vi "validate_position_v0.01.vi"(0 "valve Time Cluster":T1, 1 "which manipulator":T5(ring), 2 "Which Position to use for Experiment":T4(ring), 3 "data in":T2={"daq_ao 1"="Dev1/ao0", "daq_ai 1"="Dev1/ai0", "experiment day folder"=path "D:/DATA/8-27-15 save func testing/test.lvm", "Multiclamp init error"=0, "Multiclamp Handle Out"=0, "sampling rate (Hz)"=10000, "trial name"=""}, 7 "controls array in":refnum<vi>[](array[refnum]), 9 "time to wait for solution change (min)":dbl=2.5 min=0.0 step=0.01, 11 "error in":errorcluster, 12 "common cluster":T7, 13 "individual controls in":T6) -> (4 "output cluster":T3={"daq_ao 2"="", "Duration (s)"=0.0, "Sample Freq (Hz)"=0.0, "Phase"=0.0, "Duty Cycle"=0.0, "Jump Filter Freq (Hz)"=0.0, "Number of Replicates"=1} {"Number of Replicates" min=1 max=10}, 6 "output waveform":waveform(dbl)(graph), 8 "protocol response":waveform(dbl)[](graph) caption="Memtest", 10 "control array out":refnum<vi>[](array[refnum]), 15 "error out":errorcluster)   [LabVIEW 2019]
uses:
  pipette cleaning/pressure box/cleaning_soft/controls/actuator_type.ctl
  pipette cleaning/pressure box/cleaning_soft/controls/actuator_cluster.ctl
  machine_vision/coordinate model vis/transform_properties_actuators.ctl
  machine_vision/controls/transform_cluster_actuator.ctl
  controls/NH_method.ctl
  pipette cleaning/pressure box/cleaning_soft/controls/pressure_box_type.ctl
  pipette cleaning/pressure box/cleaning_soft/controls/pressure_box_control.ctl
  multipatch/controls/multipatch_common_controls_v4.ctl
  controls/memtest_def.ctl
  multipatch/controls/multipatch_individual_controls_v5.ctl
  Controls/Data.ctl
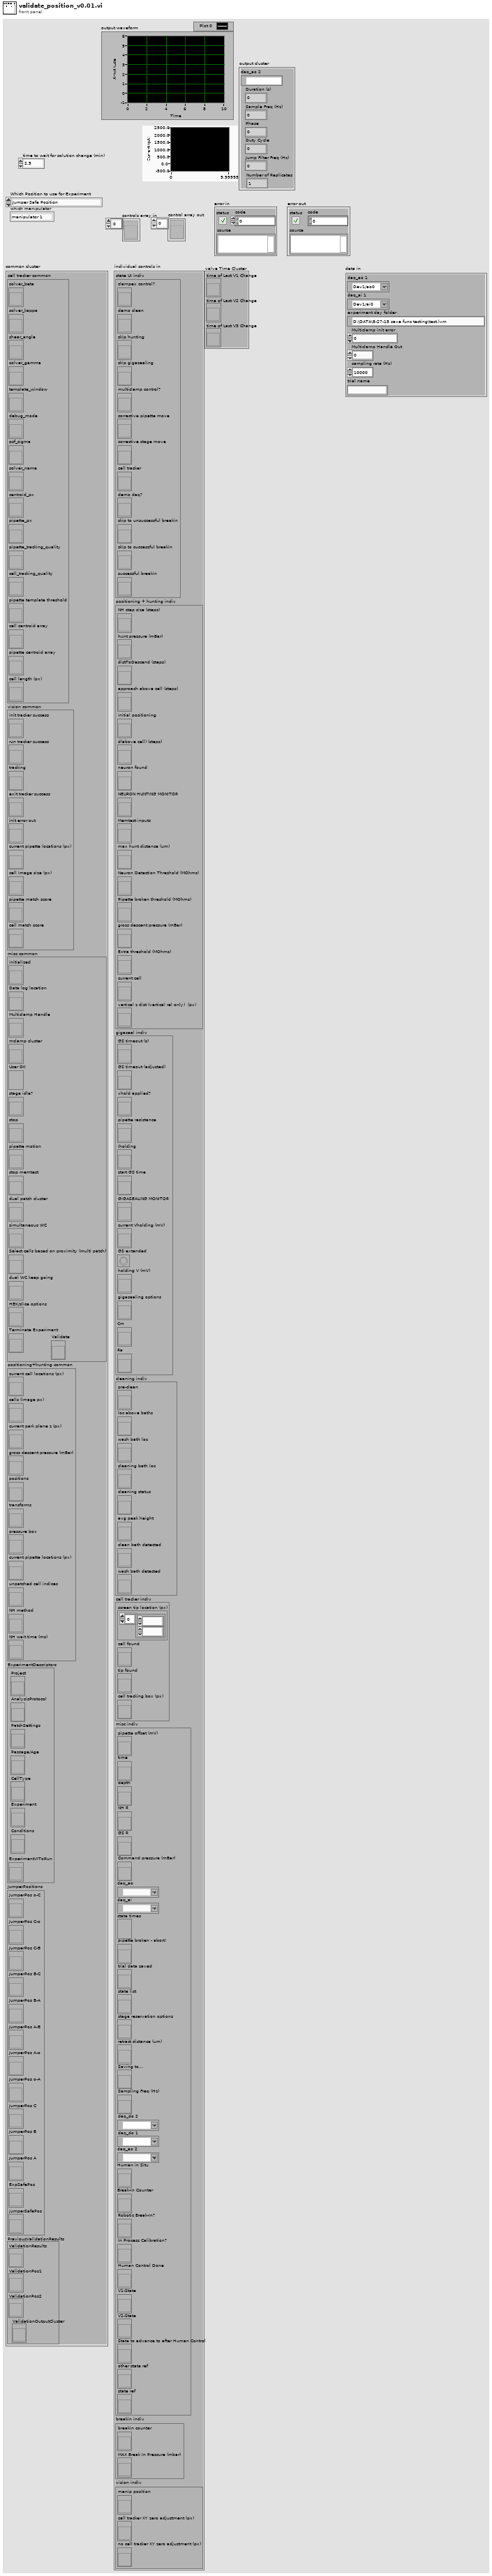
[diagram p1: front panel]
types:
  T1 = cluster{"time of Last V1 Change":refnum<vi>, "time of Last V2 Change":refnum<vi>, "time of Last V3 Change":refnum<vi>}
  T2 = typedef "Data.ctl" = cluster{"daq_ao 1":tag, "daq_ai 1":tag, "experiment day folder":path, "Multiclamp init error":i32, "Multiclamp Handle Out":u32, "sampling rate (Hz)":i32, "trial name":string}
  T3 = cluster{"daq_ao 2":tag, "Duration (s)":dbl, "Sample Freq (Hz)":dbl, "Phase":dbl, "Duty Cycle":dbl, "Jump Filter Freq (Hz)":dbl, "Number of Replicates":i16}
  T4 = enum16{"Jumper Safe Position", "Experiment Safe Position", "Jumper Position A", "Jumper Position B", "Jumper Position C", "Jumper Position o-A", "Jumper Position A-o", "Jumper Position A-B", "Jumper Position B-A", "Jumper Position B-C", "Jumper Position C-B", "Jumper Position C-o", "Jumper Position o-C"}
  T5 = enum16{"manipulator 1", "manipulator 2", "manipulator 3", "manipulator 4"}
  T6 = typedef "multipatch_individual_controls_v5.ctl" = cluster{"state UI indiv":cluster{"clampex control?":refnum<vi>, "demo clean":refnum<vi>, "skip hunting":refnum<vi>, "skip gigasealing":refnum<vi>, "multiclamp control?":refnum<vi>, "corrective pipette move":refnum<vi>, "corrective stage move":refnum<vi>, "cell tracker":refnum<vi>, "demo daq?":refnum<vi>, "skip to unsuccessful breakin":refnum<vi>, "skip to successful breakin":refnum<vi>, "successful breakin":refnum<vi>}, "positioning + hunting indiv":cluster{"NH step size (steps)":refnum<vi>, "hunt pressure (mBar)":refnum<vi>, "distToDescend (steps)":refnum<vi>, "approach above cell (steps)":refnum<vi>, "initial positioning":refnum<vi>, "d(above cell) (steps)":refnum<vi>, "neuron found":refnum<vi>, "NEURON HUNTING MONITOR":refnum<vi>, "Memtest inputs":refnum<vi>, "max hunt distance (um)":refnum<vi>, "Neuron Detection Threshold (MOhms)":refnum<vi>, "Pipette broken threshold (MOhms)":refnum<vi>, "gross descent pressure (mBar)":refnum<vi>, "Extra threshold (MOhms)":refnum<vi>, "current cell":refnum<vi>, "vertical z dist (vertical rel only)  (px)":refnum<vi>}, "gigaseal indiv":cluster{"GS timeout (s)":refnum<vi>, "GS timeout (adjusted)":refnum<vi>, "vhold applied?":refnum<vi>, "pipette resistance":refnum<vi>, "Iholding":refnum<vi>, "start GS time":refnum<vi>, "GIGASEALING MONITOR":refnum<vi>, "current Vholding (mV)":refnum<vi>, "GS extended":refnum<vi>, "holding V (mV)":refnum<vi>, "gigasealing options":refnum<vi>, "Cm":refnum<vi>, "Ra ":refnum<vi>}, "cleaning indiv":cluster{"pre-clean":refnum<vi>, "loc above baths":refnum<vi>, "wash bath loc":refnum<vi>, "cleaning bath loc":refnum<vi>, "cleaning status":refnum<vi>, "avg peak height":refnum<vi>, "clean bath detected":refnum<vi>, "wash bath detected":refnum<vi>}, "cell tracker indiv":cluster{"screen tip location (px)":refnum<vi>, "cell found":refnum<vi>, "tip found":refnum<vi>, "cell tracking box (px)":refnum<vi>}, "misc indiv":cluster{"pipette offset (mV)":refnum<vi>, "time":refnum<vi>, "depth":refnum<vi>, "NH R":refnum<vi>, "GS R":refnum<vi>, "Command pressure (mBar)":refnum<vi>, "daq_ao":tag, "daq_ai":tag, "state times":refnum<vi>, "pipette broken - abort!":refnum<vi>, "trial data saved":refnum<vi>, "state list":refnum<vi>, "stage reservation options":refnum<vi>, "retract distance (um)":refnum<vi>, "Saving to...":refnum<vi>, "Sampling Freq (Hz)":refnum<vi>, "daq_do 2":tag, "daq_do 1":tag, "daq_ao 2":tag, "Human in Situ":refnum<vi>, "Break-In Counter":refnum<vi>, "Robotic Break-In?":refnum<vi>, "In Process Calibration?":refnum<vi>, "Human Control Done":refnum<vi>, "V1-State":refnum<vi>, "V2-State":refnum<vi>, "State to advance to after Human Control":refnum<vi>, "other state ref":refnum<vi>, "state ref":refnum<vi>}, "breakin indiv":cluster{"breakin counter":refnum<vi>, "MAX Break In Pressure (mbar)":refnum<vi>}, "vision indiv":cluster{"manip position":refnum<vi>, "cell tracker XY zero adjustment (px)":refnum<vi>, "no cell tracker XY zero adjustment (px)":refnum<vi>}}
  T7 = typedef "multipatch_common_controls_v4.ctl" = cluster{"cell tracker common":cluster{"solver_beta":refnum<vi>, "solver_kappa":refnum<vi>, "shear_angle":refnum<vi>, "solver_gamma":refnum<vi>, "template_window":refnum<vi>, "debug_mode":refnum<vi>, "psf_sigma":refnum<vi>, "solver_name":refnum<vi>, "centroid_px":refnum<vi>, "pipette_px":refnum<vi>, "pipette_tracking_quality":refnum<vi>, "cell_tracking_quality":refnum<vi>, "pipette template threshold":refnum<vi>, "cell centroid array":refnum<vi>, "pipette centroid array":refnum<vi>, "cell length (px)":refnum<vi>}, "vision common":cluster{"init tracker success":refnum<vi>, "run tracker success":refnum<vi>, "tracking":refnum<vi>, "exit tracker success":refnum<vi>, "init error out":refnum<vi>, "current pipette locations (px)":refnum<vi>, "cell image size (px)":refnum<vi>, "pipette match score":refnum<vi>, "cell match score":refnum<vi>}, "misc common":cluster{"initialized":refnum<vi>, "Data log location":refnum<vi>, "Multiclamp Handle":refnum<vi>, "mclamp cluster":refnum<vi>, "User OK":refnum<vi>, "stage idle?":refnum<vi>, "stop":refnum<vi>, "pipette motion":refnum<vi>, "stop memtest":refnum<vi>, "dual patch cluster":refnum<vi>, "simultaneous WC":refnum<vi>, "Select cells based on proximity (multi patch)":refnum<vi>, "dual WC keep going":refnum<vi>, "HEK/slice options":refnum<vi>, "Terminate Experiment":refnum<vi>, "Validate":refnum<vi>}, "positioning+hunting common":cluster{"current cell locations (px)":refnum<vi>, "cells (image px)":refnum<vi>, "current park plane z (px)":refnum<vi>, "gross descent pressure (mBar)":refnum<vi>, "positions":refnum<vi>, "transforms":refnum<vi>, "pressure box":refnum<vi>, "current pipette locations (px)":refnum<vi>, "unpatched cell indices":refnum<vi>, "NH method":refnum<vi>, "NH wait time (ms)":refnum<vi>}, "ExperimentDescriptors":cluster{"Project":refnum<vi>, "AnalysisProtocol":refnum<vi>, "PatchSettings":refnum<vi>, "Passage/Age":refnum<vi>, "CellType":refnum<vi>, "Experiment":refnum<vi>, "Conditions":refnum<vi>, "ExperimentVIToRun":refnum<vi>}, "JumperPositions":cluster{"JumperPos o-C":refnum<vi>, "JumperPos C-o":refnum<vi>, "JumperPos C-B":refnum<vi>, "JumperPos B-C":refnum<vi>, "JumperPos B-A":refnum<vi>, "JumperPos A-B":refnum<vi>, "JumperPos A-o":refnum<vi>, "JumperPos o-A":refnum<vi>, "JumperPos C":refnum<vi>, "JumperPos B":refnum<vi>, "JumperPos A":refnum<vi>, "ExpSafePos":refnum<vi>, "jumperSafePos":refnum<vi>}, "PreviousValidationResults":cluster{"ValidationResults":refnum<vi>, "ValidationPos1":refnum<vi>, "ValidationPos2":refnum<vi>, "ValidationOutputCluster":refnum<vi>}}
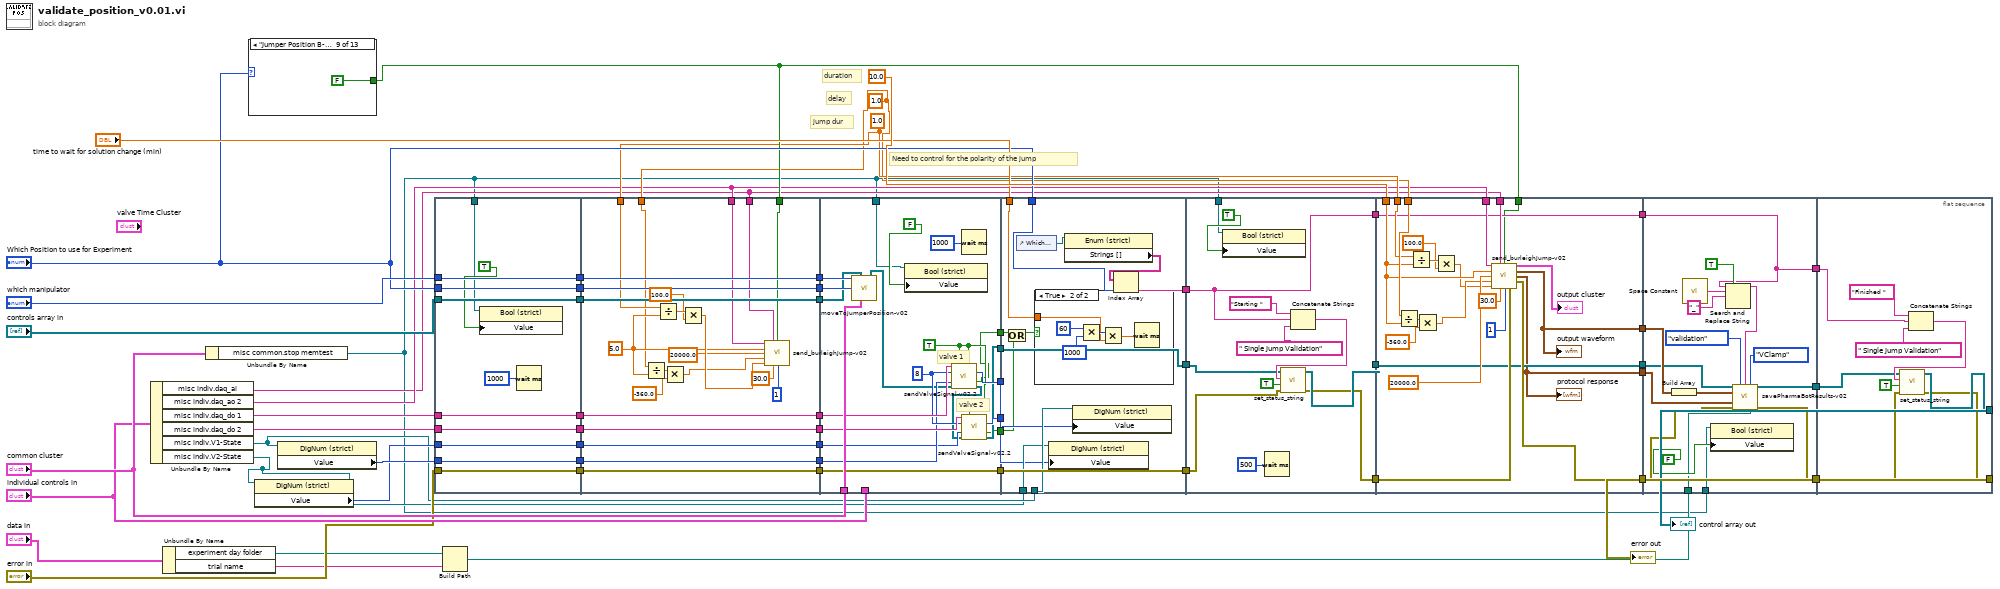
[diagram p0: block diagram]
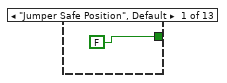
[diagram p2: hidden frame]
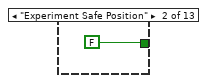
[diagram p3: hidden frame]
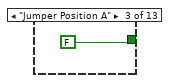
[diagram p4: hidden frame]
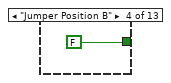
[diagram p5: hidden frame]
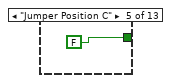
[diagram p6: hidden frame]
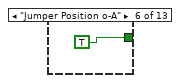
[diagram p7: hidden frame]
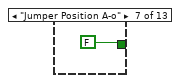
[diagram p8: hidden frame]
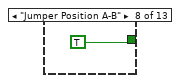
[diagram p9: hidden frame]
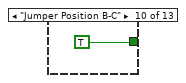
[diagram p10: hidden frame]
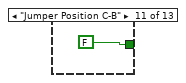
[diagram p11: hidden frame]
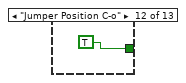
[diagram p12: hidden frame]
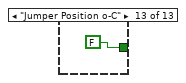
[diagram p13: hidden frame]
diagram:
  w5 = 1.0 ("Jump Duration (s)")
  w4 = 1.0 ("Jump Delay (s)")
  # "jump dur"
  # "delay"
  # "duration"
  # "Need to control for the polarity of the jump"
  n1 = Unbundle By Name("individual controls in") -> ("misc indiv.daq_ai"=w2:tag, "misc indiv.daq_ao 2"=w3:tag, "misc indiv.daq_do 1"=w59:tag, "misc indiv.daq_do 2"=w58:tag, "misc indiv.V1-State"=w49:refnum<vi>, "misc indiv.V2-State"=w48:refnum<vi>)
  n2 = Unbundle By Name("data in") -> ("experiment day folder"=w42:path, "trial name"=w41:string)
  n3 = Unbundle By Name("common cluster") -> ("misc common.stop memtest"=w1:refnum<vi>)
  n4 = case shown="\"Jumper Position B-A\"" "Which Position to use for Experiment" {
    tunnel: [FALSE FALSE FALSE FALSE FALSE TRUE FALSE TRUE FALSE TRUE FALSE TRUE FALSE] -> w6
    frame "Jumper Safe Position", Default {
    }
    frame "Experiment Safe Position" {
    }
    frame "Jumper Position A" {
    }
    frame "Jumper Position B" {
    }
    frame "Jumper Position C" {
    }
    frame "Jumper Position o-A" {
    }
    frame "Jumper Position A-o" {
    }
    frame "Jumper Position A-B" {
    }
    frame "Jumper Position B-A" {
    }
    frame "Jumper Position B-C" {
    }
    frame "Jumper Position C-B" {
    }
    frame "Jumper Position C-o" {
    }
    frame "Jumper Position o-C" {
    }
  }
  n5 = property class="DigNum (strict)"(reference=w48) -> ("Value"=w50:u16)  [unwired: 1 in, 2 out]
  n6 = property class="DigNum (strict)"(reference=w49) -> ("Value"=w51:u16)  [unwired: 1 in, 2 out]
  n7 = flat-sequence {
    tunnel: "controls array in" -> [w79]
    tunnel: w50 -> [w80]
    tunnel: w51 -> [w81]
    tunnel: "error in" -> [w82]
    tunnel: w58 -> [w83]
    tunnel: w59 -> [w84]
    tunnel: "Which Position to use for Experiment" -> [w85]
    tunnel: "which manipulator" -> [w86]
    tunnel: [w86] -> w22
    tunnel: [w85] -> w20
    tunnel: [w84] -> w18
    tunnel: [w83] -> w16
    tunnel: [w82] -> w14
    tunnel: [w81] -> w12
    tunnel: [w80] -> w10
    tunnel: [w79] -> w8
    tunnel: w1 -> [w76]
    tunnel: w22 -> [w109]
    tunnel: [w109] -> w21
    tunnel: w20 -> [w108]
    tunnel: [w108] -> w19
    tunnel: w18 -> [w107]
    tunnel: [w107] -> w17
    tunnel: w16 -> [w106]
    tunnel: [w106] -> w15
    tunnel: w14 -> [w105]
    tunnel: [w105] -> w13
    tunnel: w12 -> [w104]
    tunnel: [w104] -> w11
    tunnel: w10 -> [w103]
    tunnel: [w103] -> w9
    tunnel: w8 -> [w102]
    tunnel: [w102] -> w7
    tunnel: w6 -> [w92]
    tunnel: w5 -> [w91]
    tunnel: w4 -> [w90]
    tunnel: w3 -> [w89]
    tunnel: w2 -> [w88]
    tunnel: "common cluster" -> [w128]
    tunnel: "individual controls in" -> [_]
    tunnel: [w124] -> w53
    tunnel: [w121] -> w47
    tunnel: [w120] -> w46
    tunnel: [w116] -> w31
    tunnel: [w114] -> w26
    tunnel: [w113] -> w25
    tunnel: w21 -> [w130]
    tunnel: w19 -> [w129]
    tunnel: w17 -> [w127]
    tunnel: w15 -> [w126]
    tunnel: w13 -> [w124]
    tunnel: w11 -> [w123]
    tunnel: w9 -> [w122]
    tunnel: w7 -> [w119]
    tunnel: w1 -> [w111]
    tunnel: [w144] -> w54
    tunnel: w53 -> [w144]
    tunnel: w49 -> [w143]
    tunnel: w48 -> [w142]
    tunnel: w47 -> [w141]
    tunnel: w46 -> [w140]
    tunnel: "Which Position to use for Experiment" -> [w138]
    tunnel: [w137] -> w33
    tunnel: w31 -> [w136]
    tunnel: [w136] -> w28
    tunnel: w26 -> [w133]
    tunnel: w25 -> [w132]
    tunnel: "time to wait for solution change (min)" -> [w131]
    tunnel: w1 -> [w159]
    tunnel: [w151] -> w55
    tunnel: w54 -> [w152]
    tunnel: [w150] -> w34
    tunnel: w33 -> [w150]
    tunnel: [w153] -> w29
    tunnel: w28 -> [w154]
    tunnel: w2 -> [w181]
    tunnel: w3 -> [w180]
    tunnel: [w168] -> w56
    tunnel: w55 -> [w169]
    tunnel: [w178] -> w45
    tunnel: [w165] -> w44
    tunnel: 10.0 ("Duration (s)") -> [w170]
    tunnel: w4 -> [w173]
    tunnel: w5 -> [w172]
    tunnel: [w167] -> w35
    tunnel: w34 -> [w167]
    tunnel: [w166] -> w30
    tunnel: w29 -> [w166]
    tunnel: w6 -> [w162]
    tunnel: w1 -> [w199]
    tunnel: w56 -> [w188]
    tunnel: w45 -> [w198]
    tunnel: w44 -> [w196]
    tunnel: w40 -> [w193]
    tunnel: [w184] -> w38
    tunnel: [w187] -> w37
    tunnel: w35 -> [w185]
    tunnel: w30 -> [w186]
    tunnel: [w185] -> w27
    tunnel: [w201] -> w52
    tunnel: w38 -> [w202]
    tunnel: [w203] -> w36
    tunnel: w37 -> [w204]
    tunnel: w27 -> [w205]
    frame #0 {
      n8 = property class="Bool (strict)"(reference=w76, "Value"=TRUE ("stop memtest")) -> ()  [unwired: 1 in, 2 out]
      n9 = Wait (ms)(milliseconds to wait=u32 1000) -> ()  [unwired: 1 out]
    }
    frame #1 {
      w93 = 5.0 ("y")
      n10 = Divide(x=w90, y=w93) -> (x/y=w97:dbl)
      n11 = Divide(x=w91, y=w93) -> (x/y=w100:dbl)
      n12 = Multiply(x=w97, y=-360.0) -> (x*y=w96:dbl)
      n13 = Multiply(x=w100, y=100.0) -> (x*y=w98:dbl)
      n14 = call "send_burleighJump-v02.vi"("daq_ao 2"=w89, "daq_ai"=w88, "Jump Polarity"=w92, "Duration (s)"=w93, "Sample Freq (Hz)"=20000.0, "Phase"=w96, "Duty Cycle"=w98, "Jump Filter Freq (Hz)"=30.0, "Number of Replicates"=i16 1) -> ()  [unwired: 3 in, 4 out]
    }
    frame #2 {
      w115 = TRUE ("Set Status")
      w125 = u16 8 ("ChangeToValve")
      # "valve 2"
      # "valve 1"
      n15 = call "moveToJumperPosition-v02.vi"("which manipulator"=w130, "controls array in"=w119, "Which Jumper Position to move to?"=w129, "common cluster"=w128) -> ("control array out"=w118:refnum<vi>[])  [unwired: 10 in, 1 out]
      n16 = property class="Bool (strict)"(reference=w111, "Value"=FALSE ("stop memtest")) -> ()  [unwired: 1 in, 2 out]
      n17 = call "sendValveSignal-v02.2.vi"("daq_do"=w127, "Valve1?"=w115, "ChangeToValve"=w125, "CurrentValve"=w123, "controls array in"=w118, "Set Status"=w115) -> ("ValveSetTo"=w120:u16, "valve changed?"=w114:bool, "control array out"=w117:refnum<vi>[])  [unwired: 6 in, 1 out]
      n18 = Wait (ms)(milliseconds to wait=u32 1000) -> ()  [unwired: 1 out]
      n19 = call "sendValveSignal-v02.2.vi"("daq_do"=w126, "ChangeToValve"=w125, "CurrentValve"=w122, "controls array in"=w117, "Set Status"=w115) -> ("ValveSetTo"=w121:u16, "valve changed?"=w113:bool, "control array out"=w116:refnum<vi>[])  [unwired: 7 in, 1 out]
    }
    frame #3 {
      n20 = Or(x=w133, y=w132) -> (x .or. y?=w134:bool)
      n21 = control-ref of="Which Position to use for Experiment"() -> (w135:refnum<vi>)
      n22 = case shown="True" w134 {
        tunnel: w131 -> [_ w145]
        frame False {
        }
        frame True {
          n23 = Multiply(x=u32 60 ("milliseconds to wait"), y=u32 1000) -> (x*y=w147:u32)
          n24 = Multiply(x=w147, y=w145) -> (x*y=w146:dbl)
          n25 = Wait (ms)(milliseconds to wait=w146) -> ()  [unwired: 1 out]
        }
      }
      n26 = property class="DigNum (strict)"(reference=w142, "Value"=w141) -> ()  [unwired: 1 in, 2 out]
      n27 = property class="Enum (strict)"(reference=w135) -> ("Strings []"=w139:string[])  [unwired: 1 in, 2 out]
      n28 = property class="DigNum (strict)"(reference=w143, "Value"=w140) -> ()  [unwired: 1 in, 2 out]
      n29 = Index Array(array=w139, index=w138) -> (element=w137:string)
    }
    frame #4 {
      n30 = property class="Bool (strict)"(reference=w159, "Value"=TRUE ("stop memtest")) -> ()  [unwired: 1 in, 2 out]
      n31 = Wait (ms)(milliseconds to wait=u32 500) -> ()  [unwired: 1 out]
      n32 = Concatenate Strings("Starting " ("string"), w150, " Single Jump Validation" ("string")) -> (w157:string)
      n33 = call "set_status_string.vi"("error in"=w152, "new line?"=TRUE, "status string in"=w157, "controls array"=w154) -> ("error out"=w151:errorcluster, "controls array out"=w153:refnum<vi>[])  [unwired: 6 in]
    }
    frame #5 {
      n34 = Divide(x=w173, y=w170) -> (x/y=w174:dbl)
      n35 = Divide(x=w172, y=w170) -> (x/y=w177:dbl)
      n36 = Multiply(x=w174, y=-360.0) -> (x*y=w164:dbl)
      n37 = Multiply(x=w177, y=100.0) -> (x*y=w163:dbl)
      n38 = call "send_burleighJump-v02.vi"("daq_ao 2"=w180, "daq_ai"=w181, "Jump Polarity"=w162, "Duration (s)"=w170, "Sample Freq (Hz)"=20000.0, "Phase"=w164, "Duty Cycle"=w163, "Jump Filter Freq (Hz)"=30.0, "Number of Replicates"=i16 1, "error in"=w169) -> ("output cluster"=→"output cluster":T3, "output waveform"=w178:waveform(dbl), "protocol response"=w165:waveform(dbl)[], "error out"=w168:errorcluster)  [unwired: 2 in]
      "protocol response" <- w165
      "output waveform" <- w178
    }
    frame #6 {
      n39 = Build Array(w198) -> (w197:waveform(dbl)[])
      n40 = call <vilib>:"Space Constant.vi"() -> ("String"=w191:string)
      n41 = property class="Bool (strict)"(reference=w199, "Value"=FALSE ("stop memtest")) -> ()  [unwired: 1 in, 2 out]
      n42 = Search and Replace String(replace all?=TRUE ("replace all? (F)"), input string=w185, search string=w191, replace string="_" ("replace string (\"\")")) -> (result string=w189:string)  [unwired: 4 in, 3 out]
      n43 = call "savePharmaBotResults-v02.vi"("controls array"=w186, "protocol or memtest"=enum16{"protocol", "memtest", "validation"}."validation", "ExpPhase"=w189, "which clamp"=enum16{"VClamp", "IClamp"}."VClamp", "protocol waveform"=w197, "protocol response"=w196, "error in"=w188, "Save to (folder dir)"=w193) -> ("controls array out"=w187:refnum<vi>[], "error out"=w184:errorcluster)  [unwired: 6 in]
    }
    frame #7 {
      n44 = Concatenate Strings("Finished " ("string"), w205, " Single Jump Validation" ("string")) -> (w208:string)
      n45 = call "set_status_string.vi"("error in"=w202, "new line?"=TRUE, "status string in"=w208, "controls array"=w204) -> ("error out"=w201:errorcluster, "controls array out"=w203:refnum<vi>[])  [unwired: 6 in]
    }
  }
  n46 = Build Path(base path=w42, name or relative path=w41) -> (appended path=w40:path)
  "error out" <- w52
  "control array out" <- w36
